vi "getHeight.vi"(0 "HGF_ImaqDx in":refnum<class "HGF_ImaqDx.lvclass">, 5 "error in (no error)":errorcluster) -> (14 "HGF_ImaqDx out":refnum<class "HGF_ImaqDx.lvclass">, 17 "Height":i32, 19 "error out":errorcluster)   [LabVIEW 2014, in "HGF_IMAQ.lvlib" / "HGF_ImaqDx.lvclass"]
doc: "Returns the height of the image taken by the camera."
uses:
  HGF_ImaqDx.lvclass
  <resource>/objmgr/imaqdx.rc
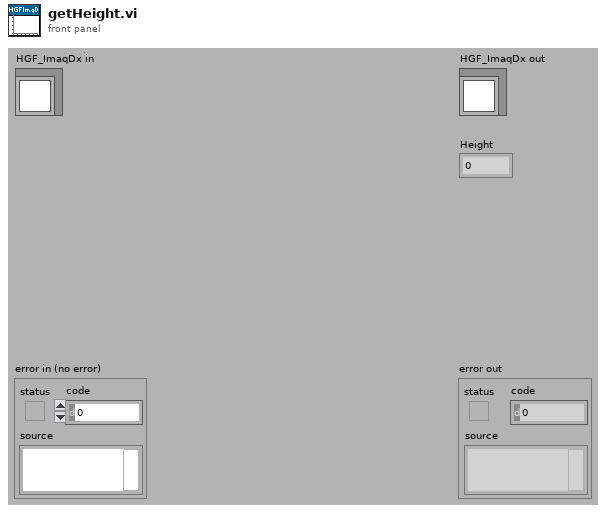
[diagram p1: front panel]
types:
  T1 = typedef "IMAQdx.ctl" = refnum<k21>
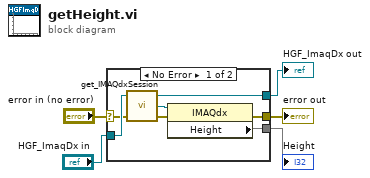
[diagram p0: block diagram]
diagram:
  n1 = case shown="No Error" "error in (no error)" {
    selector: "error in (no error)" -> [w6 w13]
    tunnel: "HGF_ImaqDx in" -> [w12 w14]
    tunnel: [w9 w14] -> w4
    tunnel: [w8 w13] -> w3
    tunnel: [w7 _] -> w2
    frame No Error {
      n2 = call "get_IMAQdxSession.vi"("error in (no error)"=w6, "HGF_ImaqDx in"=w12) -> ("error out"=w10:errorcluster, "IMAQdx Session"=w11:T1, "HGF_ImaqDx out"=w9:refnum<class "HGF_ImaqDx.lvclass">)  [unwired: 1 in]
      n3 = property class="IMAQdx"(reference=w11, error in=w10) -> (error out=w8:errorcluster, "Height"=w7)  [unwired: 1 out]
    }
    frame Error {
    }
  }
  "error out" <- w3
  "HGF_ImaqDx out" <- w4
  "Height" <- w2
